vi "Test Read Enums.vi"(11 "TwinCAT ADS in":refnum<class "TwinCAT ADS.lvclass">) -> (3 "TwinCAT ADS out":refnum<class "TwinCAT ADS.lvclass">)   [LabVIEW 2018]
uses:
  TwinCAT ADS Class/TwinCAT ADS.lvclass
  Controls/Enum.ctl
  0e82c4fa-873b-4361-ac99-2e6e4b7cd392.vi
  da0f88be-82f8-4e5b-86e7-5baa69d9b51e.vi
  4782b519-43e7-4b8e-bd72-e209be860882.vi
  e7a7b24b-aede-49d7-b369-bb451e1de87e.vi
  TwinCAT ADS Class/VIs/Data/Read.vi
  <vilib>/addons/_JKI Toolkits/Caraya/classes/Assert/Assert Equal Value_Variant.vi
  <vilib>/addons/_JKI Toolkits/Caraya/classes/Assert/Assert.lvclass
  <vilib>/addons/_JKI Toolkits/Caraya/classes/Test/Test.lvclass
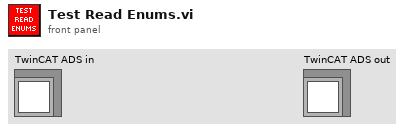
[diagram p1: front panel]
types:
  T1 = typedef "Enum.ctl" = enum16{"Member 0", "Member 1", "Member 2"}
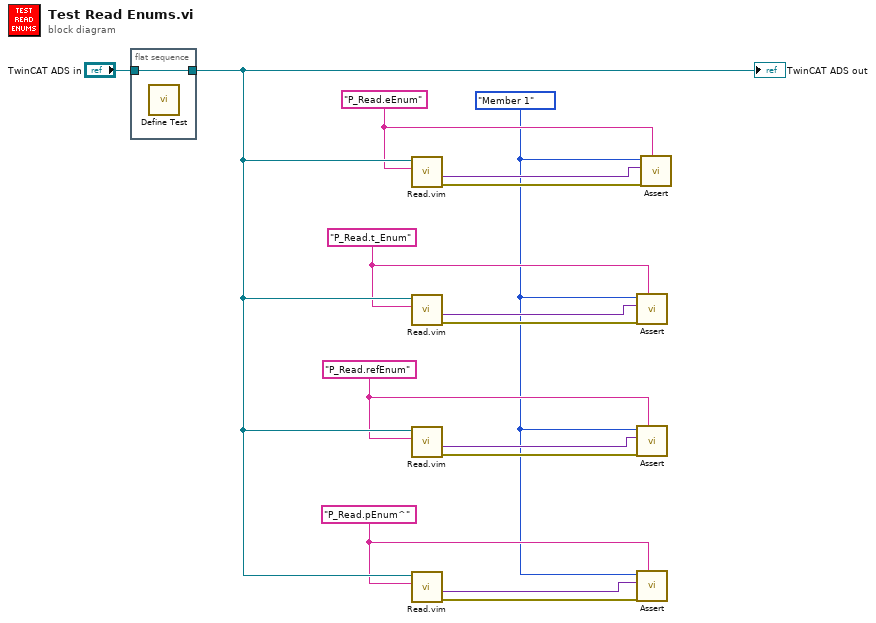
[diagram p0: block diagram]
diagram:
  w1 = Enum."Member 1"
  w7 = "P_Read.pEnum^" ("Symbol Name")
  w8 = "P_Read.refEnum" ("Symbol Name")
  w11 = "P_Read.t_Enum" ("Symbol Name")
  w12 = "P_Read.eEnum" ("Symbol Name")
  n1 = flat-sequence {
    tunnel: "TwinCAT ADS in" -> [w16]
    tunnel: [w16] -> w15
    frame #0 {
      n2 = call <vilib>:"Define Test.vi"() -> ()  [unwired: 10 in, 2 out]
    }
  }
  n3 = call "Read.vim"("Symbol Name"=w12, "TwinCAT ADS in"=w15) -> ("error out"=w14:errorcluster, "Value"=w2:variant)  [unwired: 7 in, 1 out]
  n4 = call "Read.vim"("Symbol Name"=w11, "TwinCAT ADS in"=w15) -> ("error out"=w10:errorcluster, "Value"=w3:variant)  [unwired: 7 in, 1 out]
  n5 = call "Read.vim"("Symbol Name"=w8, "TwinCAT ADS in"=w15) -> ("error out"=w9:errorcluster, "Value"=w4:variant)  [unwired: 7 in, 1 out]
  n6 = call "Read.vim"("Symbol Name"=w7, "TwinCAT ADS in"=w15) -> ("error out"=w6:errorcluster, "Value"=w5:variant)  [unwired: 7 in, 1 out]
  n7 = call-poly <vilib>:"Assert.vi"("Label"=w11, "error in (no error)"=w10, "Y"=w3, "X"=w1) -> ()  [unwired: 6 in, 2 out]
  n8 = call-poly <vilib>:"Assert.vi"("Label"=w8, "error in (no error)"=w9, "Y"=w4, "X"=w1) -> ()  [unwired: 6 in, 2 out]
  n9 = call-poly <vilib>:"Assert.vi"("Label"=w7, "error in (no error)"=w6, "Y"=w5, "X"=w1) -> ()  [unwired: 6 in, 2 out]
  n10 = call-poly <vilib>:"Assert.vi"("Label"=w12, "error in (no error)"=w14, "Y"=w2, "X"=w1) -> ()  [unwired: 6 in, 2 out]
  "TwinCAT ADS out" <- w15
